vi "Create Plugin.vi"(7 "Configuration Entry":string, 8 "error in (no error)":errorcluster, 11 "Configuration Parameters":string[](array[string])) -> (0 "error out":errorcluster, 2 "Logic Entry":T1, 3 "Configuration Entry":T1)   [LabVIEW 2021, in "Python Orchestration.lvlib"]
uses:
  Python Orchestration.lvlib
  Typedef/Scripted Line.ctl
  <vilib>/CIF Foundation/CIF Core/CIFCore/Common/Typedef/Errors.ctl
  <vilib>/CIF Foundation/CIF Utilities/Errors/Append Error Location.vi
  <vilib>/CIF Foundation/CIF Core/CIFCore/Common/CIFCoreCommon.lvlib
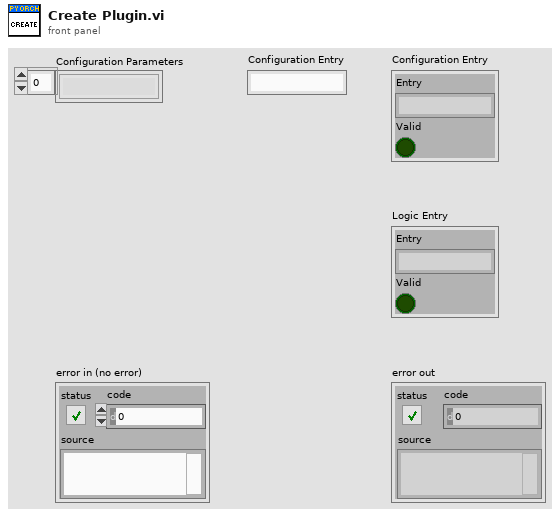
[diagram p1: front panel]
types:
  T1 = typedef "Python Orchestration.lvlib/Scripted Line.ctl" = cluster{"Entry":string, "Valid":bool}
  T2 = typedef "CIFCoreCommon.lvlib/Errors.ctl" = enum16{"Invalid Clock ID", "Long Sleep", "gRPC Server Not Found", "Config Parse", "Timestamp Wrap", "Delayed Execution", "Duplicate Channel", "Missing Channel", "Incorrect Type", "Flatten Error", "Unflatten Data", "Unique Name", "Plugin Not Found", "Plugin Type Not Found", "Plugin Version Not Found", "Manager Not Found", "Numerical Issue", "Time Jump", "Clock ID Match", "Channel Length", "Plugin Connection", "gRPC Server Connection", "PPL Name Match", "Build", "Config Log Parse", "Plugin Load", "UI Subpanel Load", "Python Name", "Invalid Name", "Unable to Change Ch Buffer", "Failed Kill", "Failed SysExec", "Function Not Implemented", "Load Timeout"}
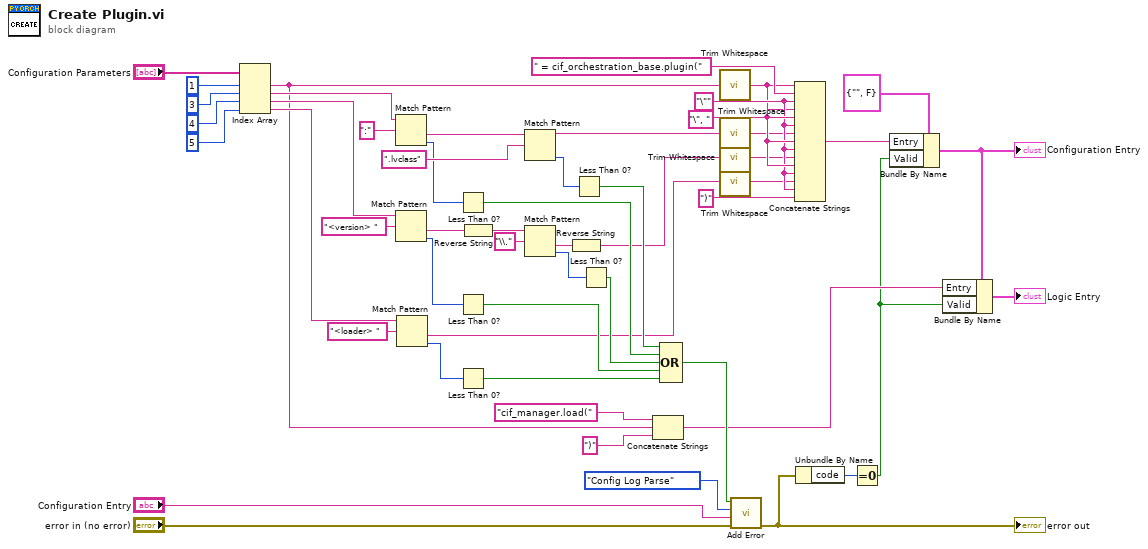
[diagram p0: block diagram]
diagram:
  w11 = "\", "
  w10 = "\""
  n1 = Index Array(array="Configuration Parameters", index #1=1 ("index"), index #2=3 ("index"), index #3=4 ("index"), index #4=5 ("index")) -> (element #1=w8:string, element #2=w35:string, element #3=w45:string, element #4=w13:string)
  n2 = Match Pattern(string=w35, regular expression=":") -> (after substring=w48:string, offset past match=w39:i32)  [unwired: 1 in, 2 out]
  n3 = Match Pattern(string=w45, regular expression="<version> ") -> (after substring=w43:string, offset past match=w37:i32)  [unwired: 1 in, 2 out]
  n4 = Match Pattern(string=w13, regular expression="<loader> ") -> (after substring=w1:string, offset past match=w15:i32)  [unwired: 1 in, 2 out]
  n5 = Less Than 0?(x=w39) -> (x < 0?=w32:bool)
  n6 = Less Than 0?(x=w37) -> (x < 0?=w34:bool)
  n7 = Less Than 0?(x=w15) -> (x < 0?=w12:bool)
  n8 = Reverse String(1:w43) -> (0:w42:string)
  n9 = Match Pattern(string=w48, regular expression=".lvclass") -> (before substring=w6:string, offset past match=w38:i32)  [unwired: 1 in, 2 out]
  n10 = Match Pattern(string=w42, regular expression="\\.") -> (after substring=w40:string, offset past match=w36:i32)  [unwired: 1 in, 2 out]
  n11 = Reverse String(1:w40) -> (0:w3:string)
  n12 = Less Than 0?(x=w38) -> (x < 0?=w31:bool)
  n13 = Less Than 0?(x=w36) -> (x < 0?=w33:bool)
  n14 = Concatenate Strings("cif_manager.load(", w8, ")" ("string")) -> (w23:string)
  n15 = Compound Arithmetic op=OR(w31, w32, w33, w34, w12) -> (w30:bool)
  n16 = call <vilib>:"Trim Whitespace.vi"("string"=w8) -> ("trimmed string"=w7:string)  [unwired: 1 in]
  n17 = call <vilib>:"Trim Whitespace.vi"("string"=w6) -> ("trimmed string"=w5:string)  [unwired: 1 in]
  n18 = call <vilib>:"Trim Whitespace.vi"("string"=w3) -> ("trimmed string"=w2:string)  [unwired: 1 in]
  n19 = call <vilib>:"Trim Whitespace.vi"("string"=w1) -> ("trimmed string"=w4:string)  [unwired: 1 in]
  n20 = call <vilib>:"Add Error.vi"("error in (no error)"="error in (no error)", "String to Append"="Configuration Entry", "Error"=Errors."Config Log Parse", "Insert Error"=w30) -> ("error out"=w25:errorcluster)  [unwired: 7 in]
  "error out" <- w25
  n21 = Concatenate Strings(w7, " = cif_orchestration_base.plugin(", w10, w7, w11, w10, w5, w11, w10, w2, w11, w10, w4, w10, ")" ("string")) -> (w26:string)
  n22 = Unbundle By Name(w25) -> ("code"=w24:i32)
  n23 = Equal To 0?(x=w24) -> (x = 0?=w22:bool)
  n24 = Bundle By Name(cluster=T1 {"Entry"="", "Valid"=FALSE} ("Logic Entry"), "Entry"=w26, "Valid"=w22) -> (w19:T1)
  "Configuration Entry" <- w19
  n25 = Bundle By Name(cluster=w19, "Entry"=w23, "Valid"=w22) -> (→"Logic Entry":T1)
